vi "Stoppani File Read.vi"(0 "String in":path) -> (3 "run":cluster{"Sampling rate":dbl, "npts":dbl}, 4 "Waveform Graph":T1(graph), 5 "Header Info":T2={"TFRFHeader"={"index"=22, "Xr"=294.1319931548027, "Yr"=349.0, "XActual"=294.1319931548027, "YActual"=349.0}, "Frequency Axis"={"Hz Resolution"=0.67291259765625, "Start Freq"=24.89776611328125, "End Freq"=3500.4913330078125}, "TSingleArray"={"fComplex"=1, "fLength"=5166.0, "a[2]"=0.0, "fConditionCheck"=1.0, "Precision"=0.0, "MtxVecVersion"=420.0, "SizeOf(TSample)"=8.0, "Tag"=0.0, "MtxVecFileCode"=64019.0, "a[9]"=0.0, "a[10]"=0.0}, "caption"="\u0000\u0000\u0000\u0000"}, 6 "Complex FRF":cluster{"t0":dbl, "dt":dbl, "Y":cdb[]})   [LabVIEW 2022 SP3]
panel:
  out "coherence":T1(graph)
  out "rest of string":string
  out "String out":string
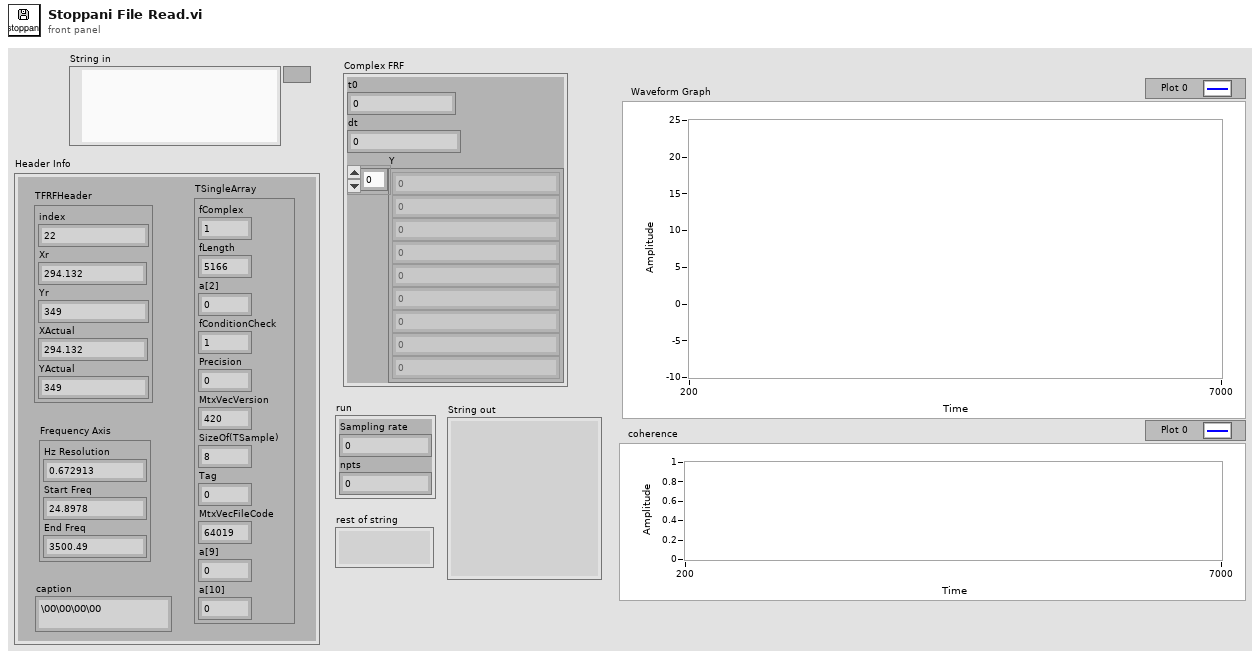
[diagram p1: front panel]
types:
  T1 = cluster{"Start freq":dbl, "Hz resolution":dbl, dbl[]}
  T2 = cluster{"TFRFHeader":cluster{"index":u32, "Xr":dbl, "Yr":dbl, "XActual":dbl, "YActual":dbl}, "Frequency Axis":cluster{"Hz Resolution":dbl, "Start Freq":dbl, "End Freq":dbl}, "TSingleArray":cluster{"fComplex":u32, "fLength":dbl, "a[2]":dbl, "fConditionCheck":dbl, "Precision":dbl, "MtxVecVersion":dbl, "SizeOf(TSample)":dbl, "Tag":dbl, "MtxVecFileCode":dbl, "a[9]":dbl, "a[10]":dbl}, "caption":string}
  T3 = enum16{"big-endian, network order", "native, host order", "little-endian"}
  T4 = cluster{"[0]":dbl, "[1]":dbl, "[2]":dbl, "[3]":dbl, "[4]":dbl}
  T5 = cluster{"[0]":sgl, "[1]":sgl, "[2]":sgl, "[3]":sgl, "[4]":sgl, "[5]":sgl, "[6]":sgl, "[7]":sgl, "[8]":sgl, "[9]":sgl, "[10]":sgl}
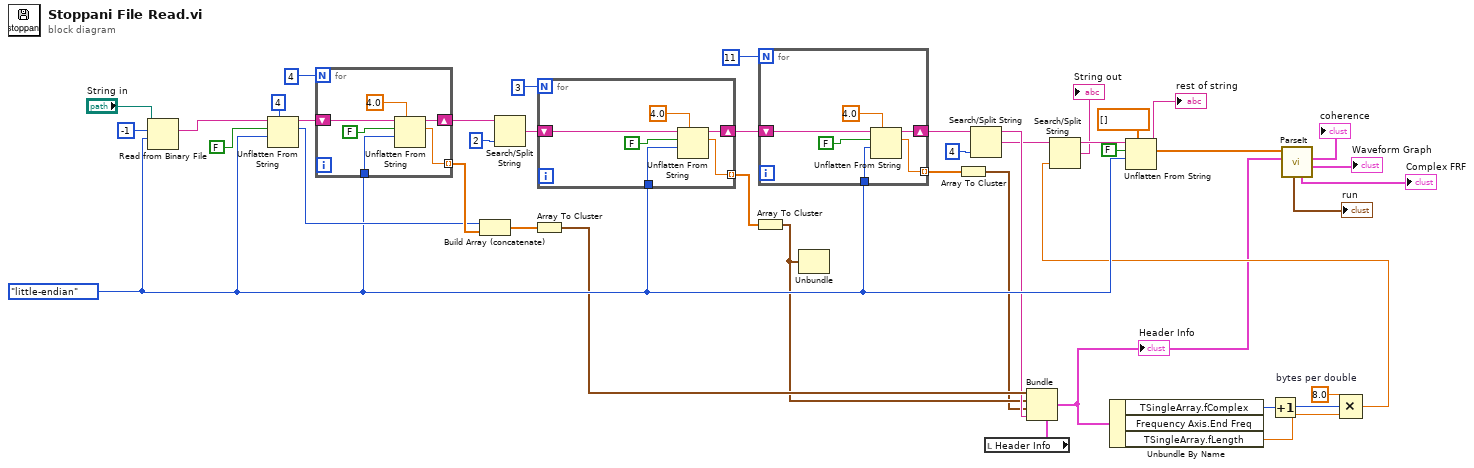
[diagram p0: block diagram]
diagram:
  w10 = 8.0  # bytes per double
  w22 = T3."little-endian" ("byte order (0:big-endian, network order)")
  n1 = Read from Binary File(9:w22, 10:-1 ("count (1)"), 11:"String in") -> (2:w16:string)  [unwired: 3 in, 3 out]
  n2 = Unflatten From String(type=u32 4 ("count (1)"), binary string=w16, data includes array or string size? (T)=FALSE, byte order (0:big-endian, network order)=w22) -> (rest of the binary string=w29:string, value=w38:u32)  [unwired: 1 in, 1 out]
  n3 = for {
    N: 4 -> [_]
    shift-right: [w46] -> w32
    shift-left: w29 -> [w48]
    tunnel: [w45] -> w40 mode=indexing
    tunnel: w22 -> [w44]
    n4 = Unflatten From String(type=4.0 ("count (1)"), binary string=w48, data includes array or string size? (T)=FALSE, byte order (0:big-endian, network order)=w44) -> (rest of the binary string=w46:string, value=w45:dbl)  [unwired: 1 in, 1 out]
  }
  n5 = Build Array (concatenate)(w38, w40) -> (w41:dbl[])
  n6 = Search/Split String(string=w32, offset (0)=2) -> (match + rest of string=w33:string)  [unwired: 1 in, 2 out]
  n7 = Array To Cluster(array=w41) -> (cluster=w21:T4)
  n8 = for {
    N: 3 -> [_]
    shift-right: [w52] -> w35
    shift-left: w33 -> [w54]
    tunnel: [w51] -> w42 mode=indexing
    tunnel: w22 -> [w50]
    n9 = Unflatten From String(type=4.0 ("count (1)"), binary string=w54, data includes array or string size? (T)=FALSE, byte order (0:big-endian, network order)=w50) -> (rest of the binary string=w52:string, value=w51:dbl)  [unwired: 1 in, 1 out]
  }
  n10 = Array To Cluster(array=w42) -> (cluster=w19:cluster{"[0]":dbl, "[1]":dbl, "[2]":dbl})
  n11 = for {
    N: 11 -> [_]
    shift-right: [w58] -> w37
    shift-left: w35 -> [w60]
    tunnel: [w57] -> w43 mode=indexing
    tunnel: w22 -> [w56]
    n12 = Unflatten From String(type=sgl 4.0 ("count (1)"), binary string=w60, data includes array or string size? (T)=FALSE, byte order (0:big-endian, network order)=w56) -> (rest of the binary string=w58:string, value=w57:sgl)  [unwired: 1 in, 1 out]
  }
  n13 = Unbundle(w19) -> ()  [unwired: 3 out]
  n14 = Array To Cluster(array=w43) -> (cluster=w18:T5)
  n15 = Search/Split String(string=w37, offset (0)=4) -> (substring before match=w20:string, match + rest of string=w15:string)  [unwired: 1 in, 1 out]
  n16 = local read "Header Info"() -> (w17:T2)
  n17 = Bundle(cluster=w17, "TFRFHeader"=w21, "Frequency Axis"=w19, "TSingleArray"=w18, "caption"=w20) -> (w1:T2)
  "Header Info" <- w1
  n18 = Unbundle By Name(w1) -> ("TSingleArray.fComplex"=w11:u32, "TSingleArray.fLength"=w9:dbl)  [unwired: 1 out]
  n19 = Increment(x=w11) -> (x+1=w8:u32)
  n20 = Compound Arithmetic op=MULTIPLY(w10, w8, w9) -> (w2:dbl)
  n21 = Search/Split String(string=w15, offset (0)=w2) -> (substring before match=w14:string, match + rest of string=→"String out":string)  [unwired: 1 in, 1 out]
  n22 = Unflatten From String(type=dbl[] [], binary string=w14, data includes array or string size? (T)=FALSE, byte order (0:big-endian, network order)=w22) -> (rest of the binary string=→"rest of string":string, value=w7:dbl[])  [unwired: 1 in, 1 out]
  n23 = call "ParseIt.vi"("Header Info"=w1, "Array"=w7) -> ("Waveform Graph"=→"Waveform Graph":T1, "coherence"=→"coherence":T1, "Complex FRF"=→"Complex FRF":cluster{"t0":dbl, "dt":dbl, "Y":cdb[]}, "run"=→"run":cluster{"Sampling rate":dbl, "npts":dbl})  [unwired: 4 in, 2 out]
